vi "Wise Drive.vi"(8 "error in":errorcluster, 11 "Joystick Control":dbl) -> (0 "error out":errorcluster, 3 "Throttle":dbl)   [LabVIEW 2016]
panel:
  in  "Low slope":dbl=0.5
  in  "Switch value":dbl=0.7
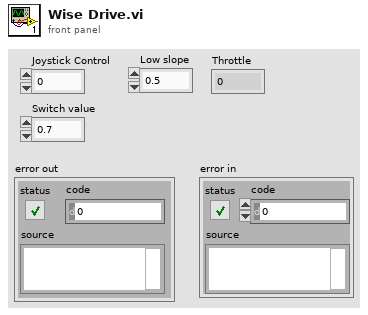
[diagram p1: front panel]
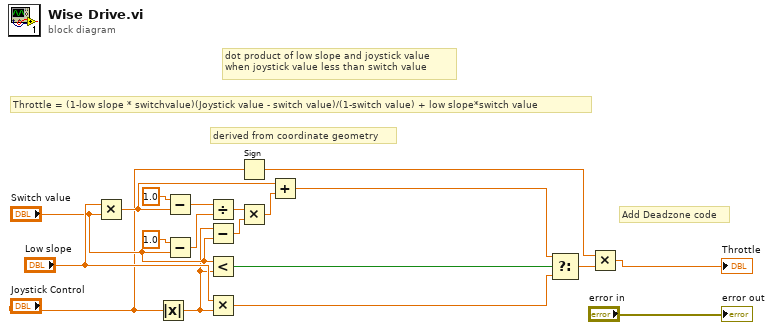
[diagram p0: block diagram]
diagram:
  # "Add Deadzone code"
  # "derived from coordinate geometry"
  # "Throttle = (1-low slope * switchvalue)(Joystick value - switch value)/(1-switch value) + low slope*switch value"
  # "dot product of low slope and joystick value \nwhen joystick value less than switch value"
  n1 = Multiply(x="Low slope", y="Switch value") -> (x*y=w15:dbl)
  n2 = Absolute Value(x="Joystick Control") -> (abs(x)=w6:dbl)
  n3 = Subtract(x=1.0, y=w15) -> (x-y=w14:dbl)
  n4 = Subtract(x=1.0, y="Switch value") -> (x-y=w12:dbl)
  n5 = Divide(x=w14, y=w12) -> (x/y=w11:dbl)
  n6 = Subtract(x=w6, y="Switch value") -> (x-y=w10:dbl)
  n7 = Less?(x="Switch value", y=w6) -> (x < y?=w18:bool)
  n8 = Multiply(x="Low slope", y=w6) -> (x*y=w19:dbl)
  n9 = Sign(1:"Joystick Control") -> (0:w5:dbl)
  n10 = Multiply(x=w11, y=w10) -> (x*y=w9:dbl)
  n11 = Add(x=w15, y=w9) -> (x+y=w17:dbl)
  n12 = Select(t=w17, s=w18, f=w19) -> (s? t:f=w4:dbl)
  n13 = Multiply(x=w5, y=w4) -> (x*y=→"Throttle":dbl)
  "error out" <- "error in"
